vi "Multi Shear Test Pause for Reconnect Case.vi"() -> ()   [LabVIEW 2013]
panel:
  in  "Forward Speed":dbl
  in  "Resume":bool
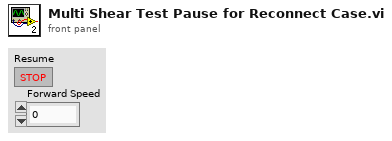
[diagram p1: front panel]
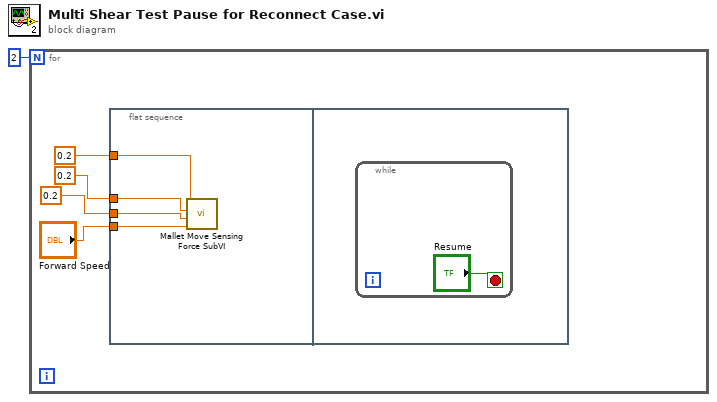
[diagram p0: block diagram]
diagram:
  n1 = for {
    N: 2 -> [_]
    n2 = flat-sequence {
      tunnel: "Forward Speed" -> [w9]
      tunnel: 0.2 ("Reverse Speed") -> [w8]
      tunnel: 0.2 ("Forward Time") -> [w7]
      tunnel: 0.2 ("Reverse Time") -> [w6]
      frame #0 {
        n3 = call "Mallet Move Sensing Force SubVI.vi"("Forward Speed"=w9, "Reverse Speed"=w8, "Forward Time"=w7, "Reverse Time"=w6) -> ()  [unwired: 6 in, 2 out]
      }
      frame #1 {
        n4 = while {
          stop <- "Resume" stop-if-true
        }
      }
    }
  }
